vi "Read Frame From TDMS.vi"(10 "Frame Number":i32, 11 "tdms file in":refnum<k34>) -> (2 "\"frame n\" string":string, 3 "tdms file out":refnum<k34>, 5 "pDataBuffer":u16[](array[numeric]))   [LabVIEW 2020]
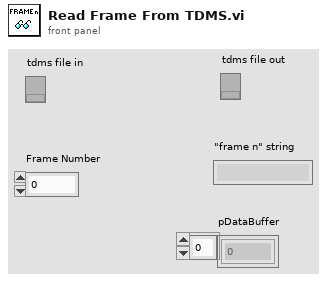
[diagram p1: front panel]
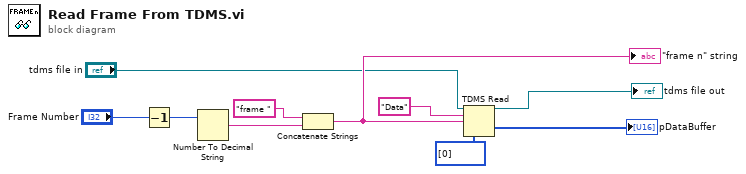
[diagram p0: block diagram]
diagram:
  n1 = Decrement(x="Frame Number") -> (x-1=w1:i32)
  n2 = Number To Decimal String(number=w1) -> (decimal integer string=w9:string)  [unwired: 1 in]
  n3 = Concatenate Strings("frame ", w9) -> (w10:string)
  "\"frame n\" string" <- w10
  n4 = TDMS Read(0:"tdms file in", 5:"Data" ("group name in (Untitled)"), 7:w10, 12:u16[] [0] ("pDataBuffer")) -> (4:→"tdms file out":refnum<k34>, 10:→"pDataBuffer":u16[])  [unwired: 4 in, 4 out]
